vi "RSZVB Get Mixer Delay Division By Two Enabled.vi"(8 "error in (no error)":errorcluster {"code" format="%.0x"}, 9 "Channel (1)":i32=1, 11 "VISA session":refnum<visa-resource-name>) -> (0 "error out":errorcluster {"code" format="%.0x"}, 2 "Division By Two":bool, 3 "dup VISA session":refnum<visa-resource-name>)   [LabVIEW 2011]
doc: "Returns the division state of loaded mixer delay calibration data by two.\n\nRemote-control command(s):\n[SENSe<Ch>:]FREQuency:MDELay:DIVide?"
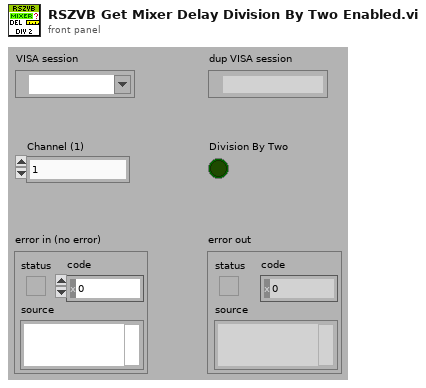
[diagram p1: front panel]
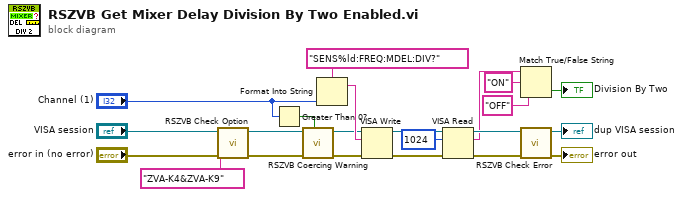
[diagram p0: block diagram]
diagram:
  n1 = call "RSZVB Check Option.vi"("error in (no error)"="error in (no error)", "Options"="ZVA-K4&ZVA-K9", "VISA session"="VISA session") -> ("error out"=w2:errorcluster, "dup VISA session"=w1:refnum<visa-resource-name>)  [unwired: 7 in]
  n2 = Greater Than 0?(x="Channel (1)") -> (x > 0?=w7:bool)
  n3 = call "RSZVB Coercing Warning.vi"("In Range?"=w7, "error in (no error)"=w2, "VISA session"=w1) -> ("error out"=w21:errorcluster, "dup VISA session"=w20:refnum<visa-resource-name>)  [unwired: 7 in]
  n4 = Format Into String(format string="SENS%ld:FREQ:MDEL:DIV?", "Channel (1)") -> (resulting string=w22:string)  [unwired: 2 in, 1 out]
  n5 = VISA Write(VISA resource name=w20, write buffer=w22, error in (no error)=w21) -> (VISA resource name out=w11:refnum<visa-resource-name>, error out=w12:errorcluster)  [unwired: 1 out]
  n6 = VISA Read(VISA resource name=w11, byte count=u32 1024, error in (no error)=w12) -> (VISA resource name out=w16:refnum<visa-resource-name>, read buffer=w15:string, error out=w17:errorcluster)  [unwired: 1 out]
  n7 = Match True/False String(2:"OFF" ("false string"), 3:"ON" ("true string"), 4:w15) -> (0:→"Division By Two":bool)  [unwired: 1 out]
  n8 = call "RSZVB Check Error.vi"("error in (no error)"=w17, "VISA session"=w16) -> ("error out"=→"error out":errorcluster, "dup VISA session"=→"dup VISA session":refnum<visa-resource-name>)  [unwired: 8 in]
